vi "DeviceNet Read Data.vi"() -> ()   [LabVIEW 2010]
uses:
  <vilib>/nidnet/Nidnet.llb/DnetIntfConfig.ctl
panel:
  in  "DeviceNet Interface Configuration":T1 {"IntfMacId" max=63 step=1}
  out "Error out":errorcluster {"code" format="%.0x"}
  in  "Error in":errorcluster {"code" format="%.0x"}
  in  "IntfName":T2(ring)
  in  "ByteOffset":u16
  out "String Out":string
  out "DBL/SGL Out":dbl format="%.2f"
  out "8[TF] Out":bool[](array[boolean])
  out "I32/I16/I8 Out":i32
  out "U32/U16/U8 Out":u32
  in  "Dnet Input Type":T3(ring)
  out "DnetData in":u8[](array[numeric])
  # "DeviceNet Read Data"
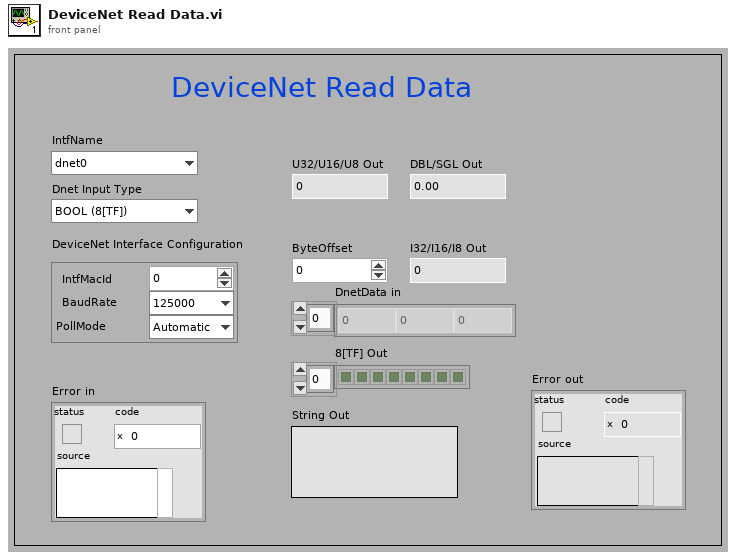
[diagram p1: front panel]
types:
  T1 = typedef "DnetIntfConfig.ctl" = cluster{"IntfMacId":u32, "BaudRate":enum32{"125000", "250000", "500000"}, "PollMode":enum32{"Automatic", "Scanned", "Individual"}}
  T2 = enum16{"dnet0", "dnet1", "dnet2", "dnet3", "dnet4", "dnet5", "dnet6", "dnet7", "dnet8", "dnet9", "dnet10", "dnet11", "dnet12", "dnet13", "dnet14", "dnet15", "dnet16", "dnet17", "dnet18", "dnet19", "dnet20", "dnet21", "dnet22", "dnet23", "dnet24", "dnet25", "dnet26", "dnet27", "dnet28", "dnet29", "dnet30", "dnet31"}
  T3 = enum16{"BOOL (8[TF])", "SINT (I8)", "INT (I16)", "DINT (I32)", "USINT (U8)", "UINT (U16)", "UDINT (U32)", "REAL (SGL)", "LREAL (DBL)", "SHORT_STRING (abc)", "STRING (abc)"}
  T4 = typedef "xobjhandle.ctl" = u32
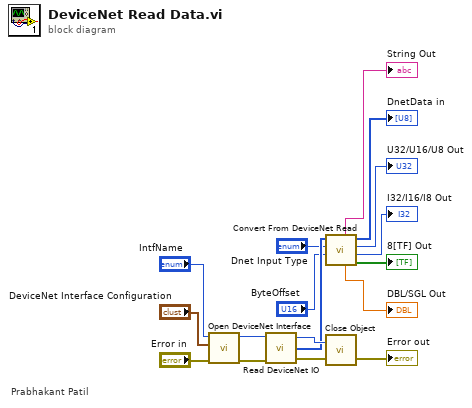
[diagram p0: block diagram]
diagram:
  # "Prabhakant Patil"
  n1 = call <vilib>:"Open DeviceNet Interface.vi"("Error in"="Error in", "DeviceNet Interface Configuration"="DeviceNet Interface Configuration", "IntfName"="IntfName") -> ("Error out"=w16:errorcluster, "ObjHandle out"=w17:T4)  [unwired: 3 in]
  n2 = call <vilib>:"Read DeviceNet IO.vi"("ObjHandle in"=w17, "Error in"=w16) -> ("ObjHandle out"=w15:T4, "Data"=w9:u8[], "Error out"=w14:errorcluster)  [unwired: 3 in]
  n3 = call <vilib>:"Convert From DeviceNet Read.vi"("ByteOffset"="ByteOffset", "DnetType"="Dnet Input Type", "DnetData in"=w9) -> ("8[TF] out"=→"8[TF] Out":bool[], "I32/I16/I8 out"=→"I32/I16/I8 Out":i32, "U32/U16/U8 out"=→"U32/U16/U8 Out":u32, "DnetData out"=→"DnetData in":u8[], "DBL/SGL out"=→"DBL/SGL Out":dbl, "abc out"=→"String Out":string)  [unwired: 3 in]
  n4 = call <vilib>:"Close Object.vi"("Error in"=w14, "ObjHandle in"=w15) -> ("Error out"=→"Error out":errorcluster)  [unwired: 1 in]
